vi "Load saved scan settings_arbitray cluster elements.vi"() -> (0 "Scan settings array":T1[](array[typedef]) {"Number of pixels to stabilize \nper substrate" items=["1", "2", "3", "4", "5", "6", "7", "8"]; "Range Options" items=["Auto Range", "Semi-Auto Range", "100 uA", "1 mA", "10 mA", "100 mA", "1A"]}, 3 "Scan settings name array":string[](array[string]), 4 "Settings folder path":path)   [LabVIEW 2011]
uses:
  Typedefs/Scan settings.ctl
  <vilib>/Utility/file.llb/Read From Spreadsheet File (string).vi
panel:
  in  "Scan settings":T1={"Light intensity (Suns)"=1.0, "Pre-bias time (s)"=0.0, "Maximum voltage (V)"=1.4, "Minimum voltage (V)"=0.01, "Range Options"=10, "1st scan FB to SC?"=TRUE, "Step Size (V)"=0.0, "Source Delay (s)"=0.0, "Inverted device"=FALSE, "Measure stabilized power output"=FALSE, "Stabilzation time (s)"=0.0, "Use Vmp from JV scan"=FALSE, "Stabization voltage (V)"=0.0, "Only stabilize best pixels"=TRUE, "Number of pixels to stabilize \nper substrate"=0, "Stabilization time step (s)"=1.0, "Use max power tracking"=FALSE, "Pre-bias voltage (V)"=-1.4, "No. of data point averages"=1.0, "No. of J-V averages"=1.0, "Integration time (ms)"=200.0} {"Number of pixels to stabilize \nper substrate" items=["1", "2", "3", "4", "5", "6", "7", "8"]; "Range Options" items=["Auto Range", "Semi-Auto Range", "100 uA", "1 mA", "10 mA", "100 mA", "1A"]}
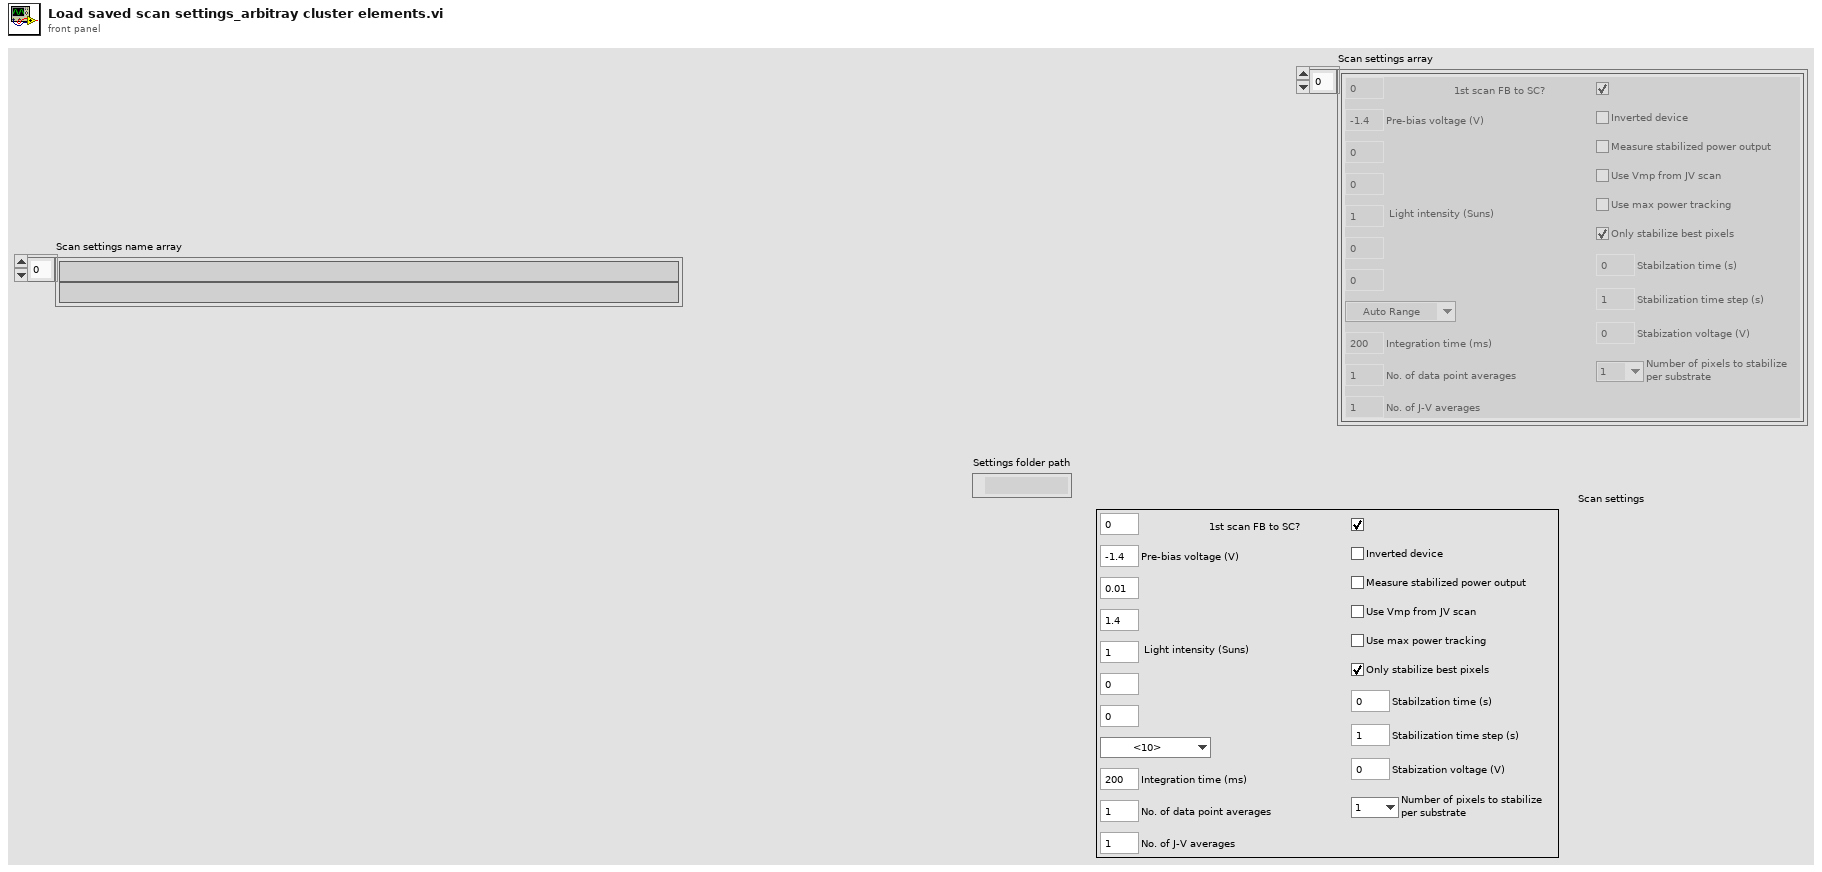
[diagram p1: front panel]
types:
  T1 = typedef "Scan settings.ctl" = cluster{"Light intensity (Suns)":dbl, "Pre-bias time (s)":dbl, "Maximum voltage (V)":dbl, "Minimum voltage (V)":dbl, "Range Options":u16, "1st scan FB to SC?":bool, "Step Size (V)":dbl, "Source Delay (s)":dbl, "Inverted device":bool, "Measure stabilized power output":bool, "Stabilzation time (s)":dbl, "Use Vmp from JV scan":bool, "Stabization voltage (V)":dbl, "Only stabilize best pixels":bool, "Number of pixels to stabilize \nper substrate":u16, "Stabilization time step (s)":dbl, "Use max power tracking":bool, "Pre-bias voltage (V)":dbl, "No. of data point averages":dbl, "No. of J-V averages":dbl, "Integration time (ms)":dbl}
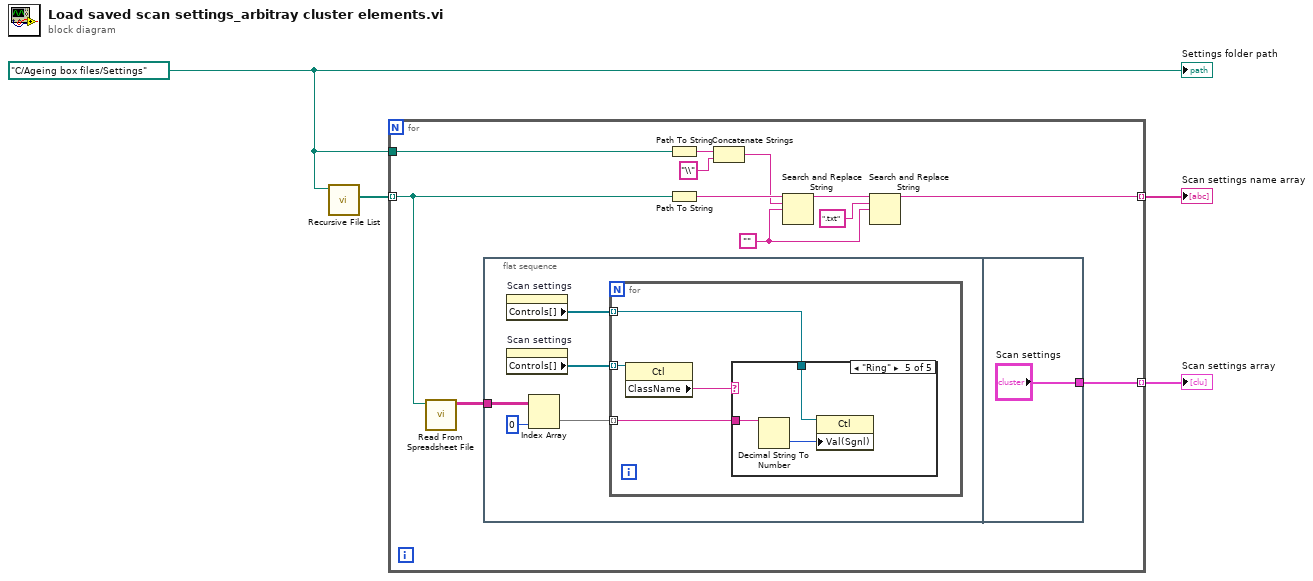
[diagram p0: block diagram]
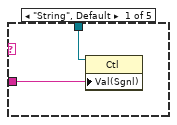
[diagram p2: hidden frame]
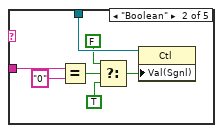
[diagram p3: hidden frame]
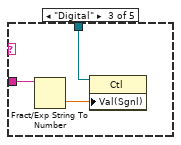
[diagram p4: hidden frame]
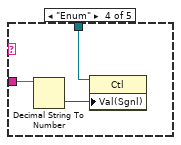
[diagram p5: hidden frame]
diagram:
  w3 = path "C:/Ageing box files/Settings"
  n1 = call <vilib>:"Recursive File List.vi"("Folder Path"=w3) -> ("All Files in Dir"=w4:path[])  [unwired: 6 in, 4 out]
  n2 = for {
    tunnel: w4 -> [w6] mode=indexing
    tunnel: w3 -> [w8]
    tunnel: [w7] -> w2 mode=indexing
    tunnel: [w5] -> w1 mode=indexing
    w14 = ""
    n3 = call-poly <vilib>:"Read From Spreadsheet File.vi"("file path (dialog if empty)"=w6) -> ("all rows"=w9:string[][])  [unwired: 6 in, 4 out]
    n4 = flat-sequence {
      tunnel: w9 -> [w19]
      tunnel: ["Scan settings"] -> w5
      frame #0 {
        n5 = property on="Scan settings" class="Clust (strict)"() -> ("Controls[]"=w20:refnum<vi>[])  [unwired: 2 in, 2 out]
        n6 = property on="Scan settings" class="Clust (strict)"() -> ("Controls[]"=w21:refnum<vi>[])  [unwired: 2 in, 2 out]
        n7 = Index Array(array=w19, index (col)=0 ("disabled index (col)")) -> (element=w17:string[])  [unwired: 1 in]
        n8 = for {
          tunnel: w21 -> [w25] mode=indexing
          tunnel: w20 -> [w23] mode=indexing
          tunnel: w17 -> [w22] mode=indexing
          n9 = property class="Ctl"(reference=w25) -> ("ClassName"=w24:string)  [unwired: 1 in, 2 out]
          n10 = case shown="\"Ring\"" w24 {
            tunnel: w23 -> [w27 w34 w37 w40 w43]
            tunnel: w22 -> [w26 w33 w36 w39 w42]
            frame "String", Default {
              n11 = property class="Ctl"(reference=w27, "Val(Sgnl)"=w26) -> ()  [unwired: 1 in, 2 out]
            }
            frame "Boolean" {
              n12 = Equal?(x=w33, y="0") -> (x = y?=w31:bool)
              n13 = Select(t=FALSE, s=w31, f=TRUE) -> (s? t:f=w28:bool)
              n14 = property class="Ctl"(reference=w34, "Val(Sgnl)"=w28) -> ()  [unwired: 1 in, 2 out]
            }
            frame "Digital" {
              n15 = Fract/Exp String To Number(string=w36) -> (number=w35:dbl)  [unwired: 3 in, 1 out]
              n16 = property class="Ctl"(reference=w37, "Val(Sgnl)"=w35) -> ()  [unwired: 1 in, 2 out]
            }
            frame "Enum" {
              n17 = Decimal String To Number(string=w39) -> (number=w38:i32)  [unwired: 2 in, 1 out]
              n18 = property class="Ctl"(reference=w40, "Val(Sgnl)"=w38) -> ()  [unwired: 1 in, 2 out]
            }
            frame "Ring" {
              n19 = Decimal String To Number(string=w42) -> (number=w41:i32)  [unwired: 2 in, 1 out]
              n20 = property class="Ctl"(reference=w43, "Val(Sgnl)"=w41) -> ()  [unwired: 1 in, 2 out]
            }
          }
        }
      }
      frame #1 {
      }
    }
    n21 = Path To String(path=w8) -> (string=w12:string)
    n22 = Path To String(path=w6) -> (string=w15:string)
    n23 = Concatenate Strings(w12, "\\") -> (w10:string)
    n24 = Search and Replace String(input string=w15, search string=w10, replace string=w14) -> (result string=w13:string)  [unwired: 5 in, 3 out]
    n25 = Search and Replace String(input string=w13, search string=".txt", replace string=w14) -> (result string=w7:string)  [unwired: 5 in, 3 out]
  }
  "Scan settings name array" <- w2
  "Scan settings array" <- w1
  "Settings folder path" <- w3
